vi "Delete old files.vi"(6 "Delete File Action":T1, 8 "error in (no error)":errorcluster, 9 "Entire hierachy (F)":bool, 10 "Retention":i32, 11 "Directory":string[](array[string])) -> (0 "error out":errorcluster)   [LabVIEW 2017, in "File.lvlib"]
uses:
  File.lvlib
  Control/Delete File Action.ctl
  Control/Parent path.ctl
  Error Handler/Error.lvlib
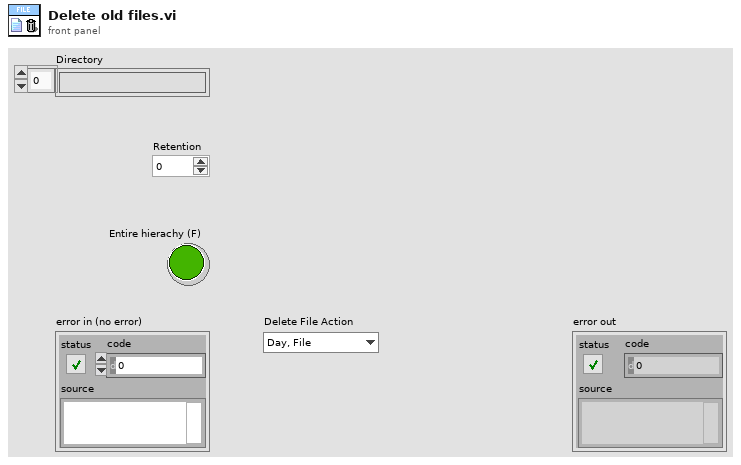
[diagram p1: front panel]
types:
  T1 = typedef "File.lvlib/Delete File Action.ctl" = enum16{"Day, File", "Day, Folder", "Month, File", "Month, Folder"}
  T2 = cluster{"Retention":i32, "Directory":string[], "Entire hierachy (F)":bool, "current time":timestamp}
  T3 = typedef "File.lvlib/Parent path.ctl" = enum16{"Project", "Setting", "Log"}
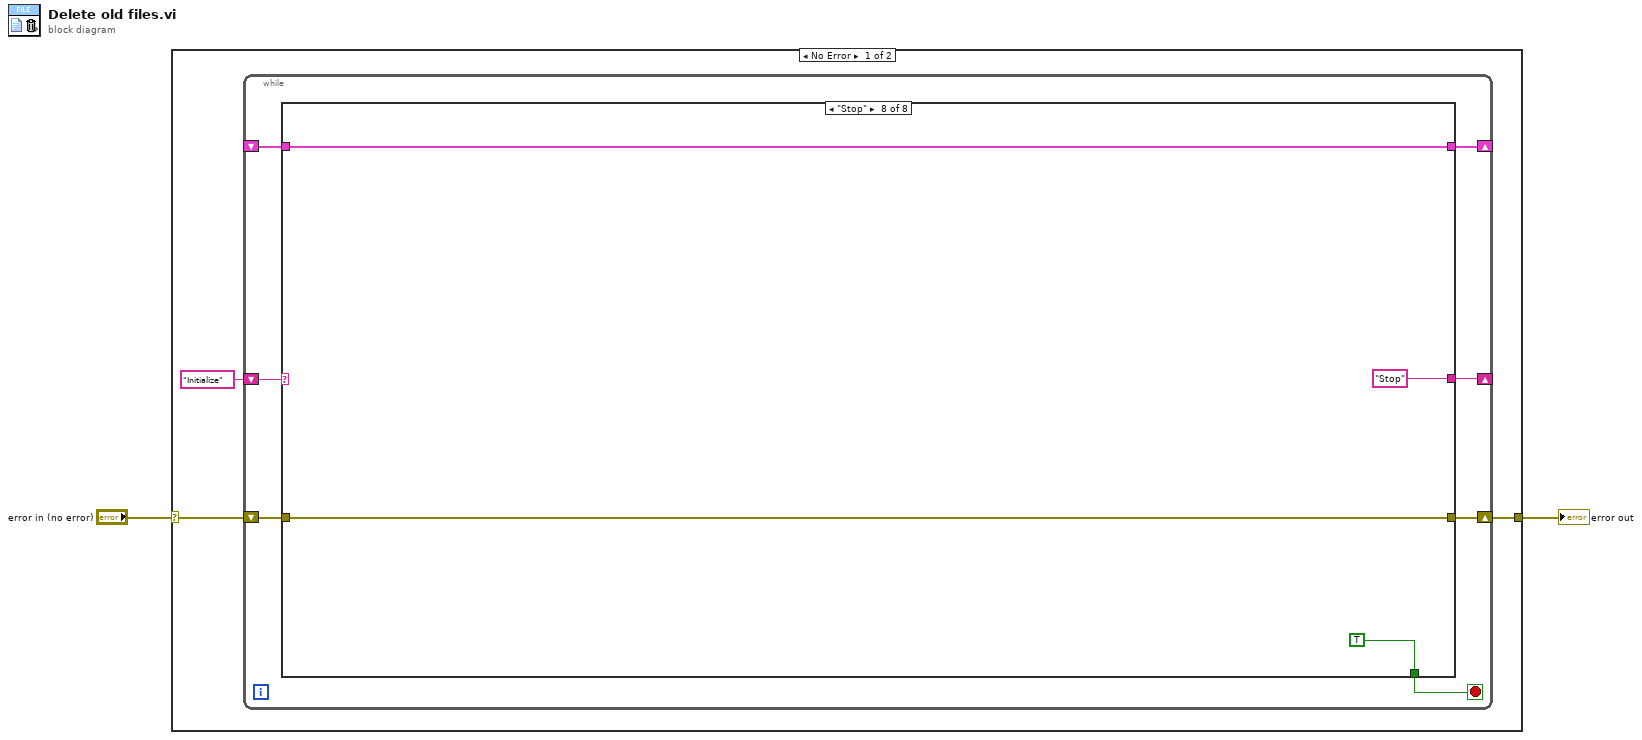
[diagram p0: block diagram]
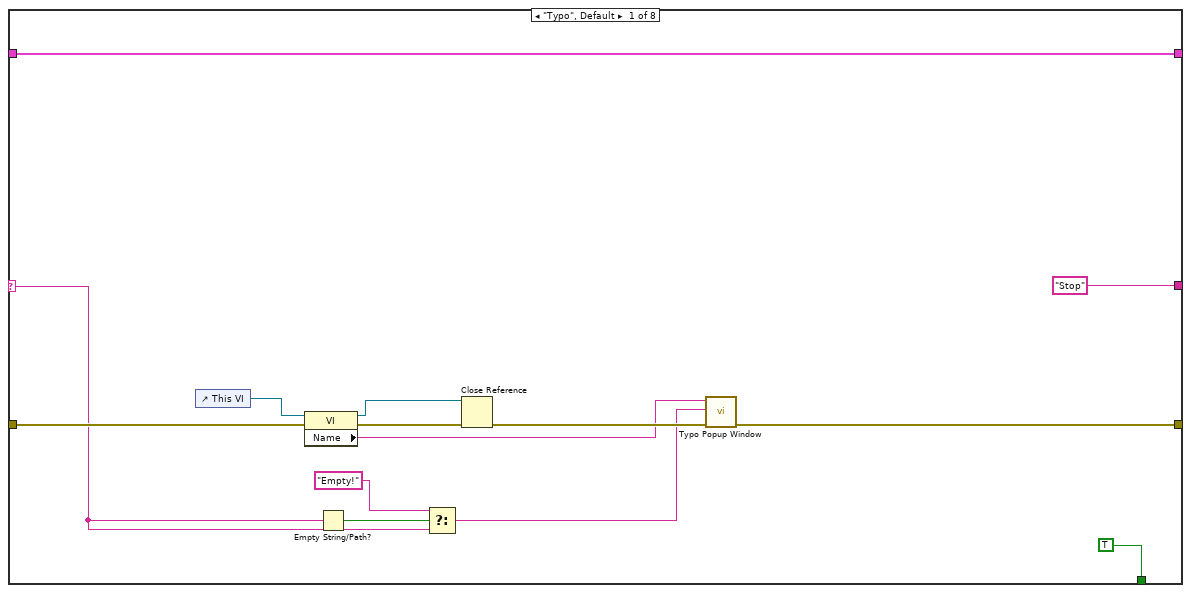
[diagram p2: hidden frame]
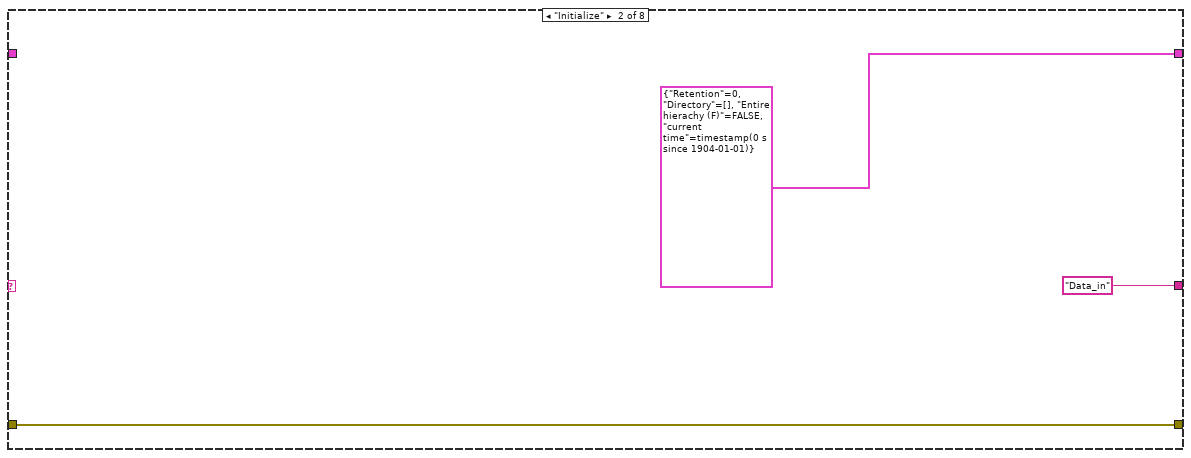
[diagram p3: hidden frame]
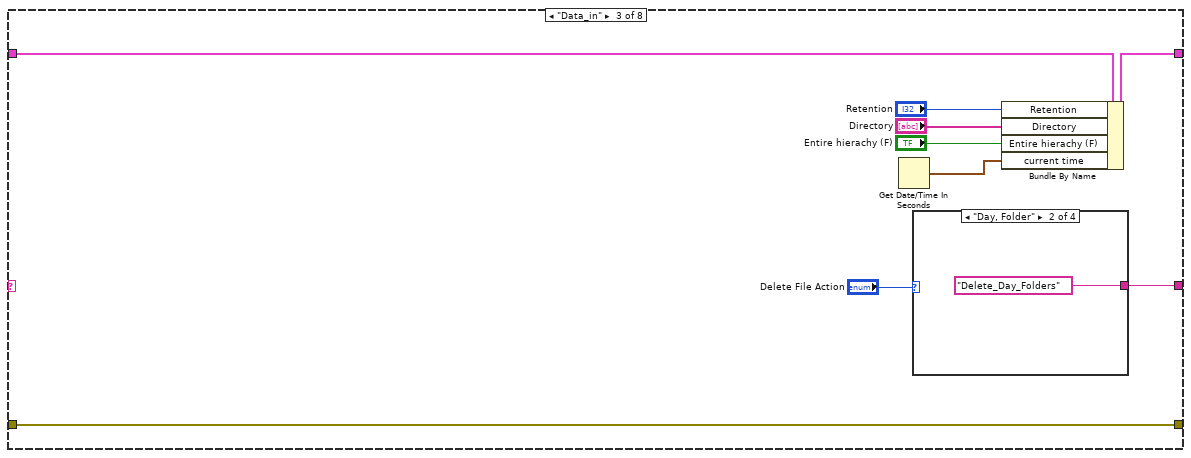
[diagram p4: hidden frame]
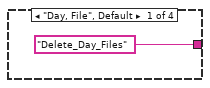
[diagram p5: hidden frame]
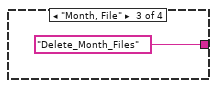
[diagram p6: hidden frame]
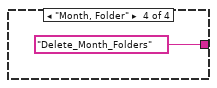
[diagram p7: hidden frame]
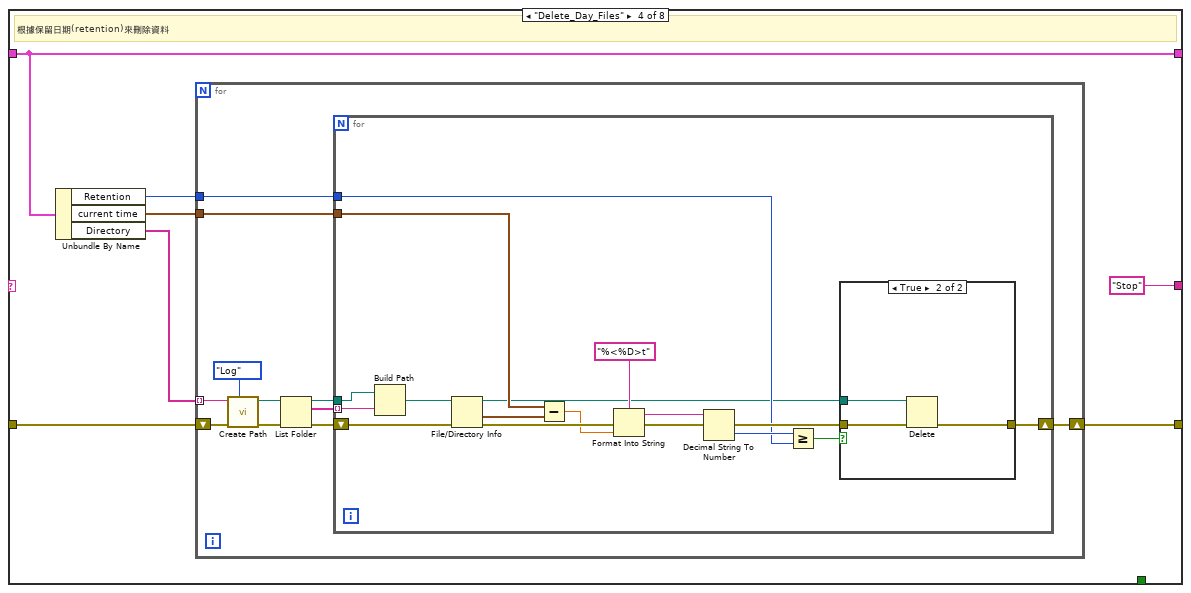
[diagram p8: hidden frame]
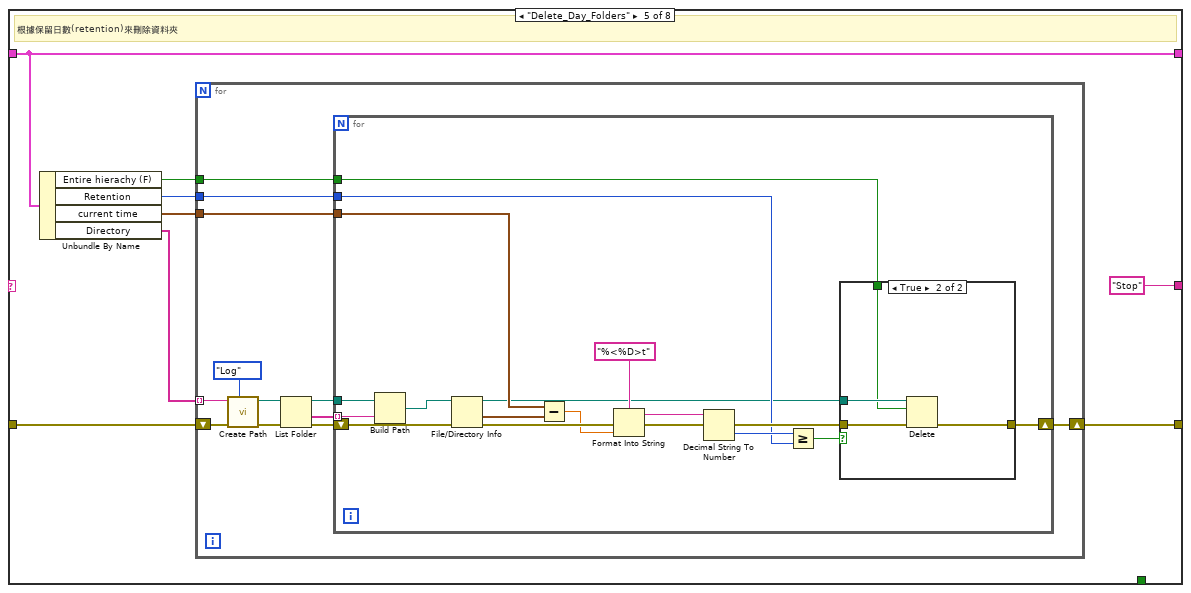
[diagram p10: hidden frame]
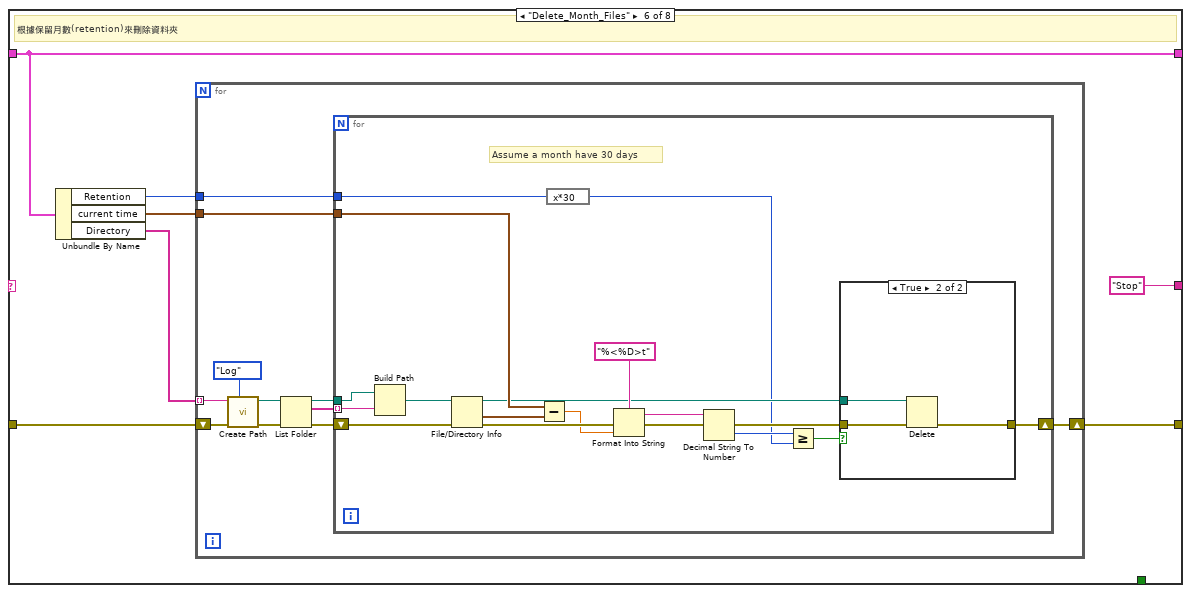
[diagram p12: hidden frame]
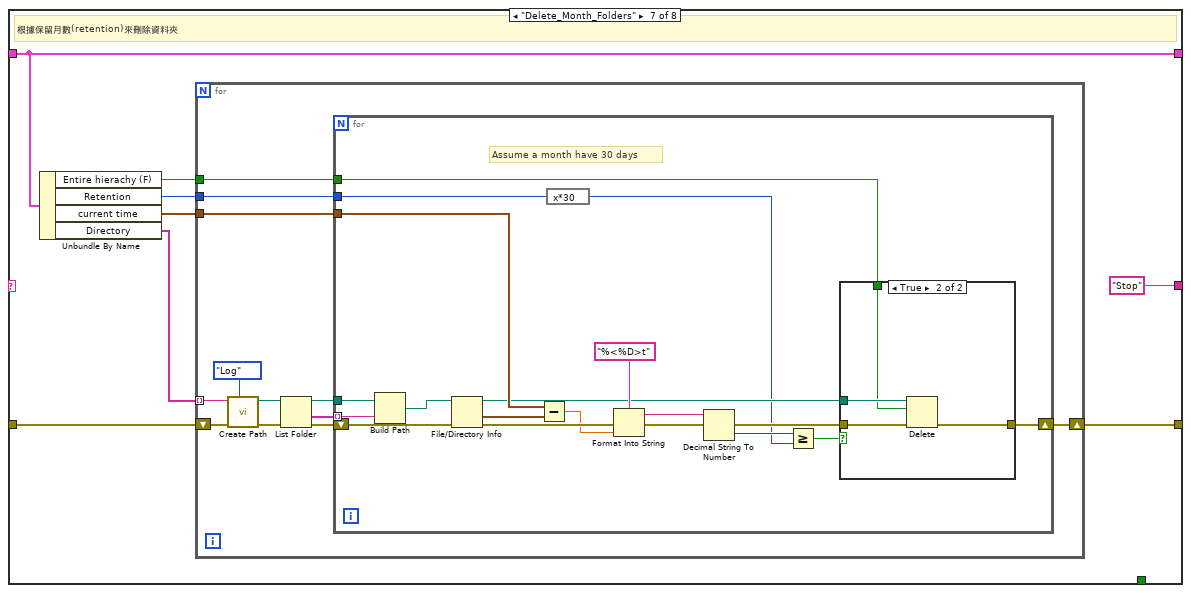
[diagram p14: hidden frame]
diagram:
  n1 = case shown="No Error" "error in (no error)" {
    selector: "error in (no error)" -> [w4 w209]
    tunnel: [w3 w209] -> w1
    frame No Error {
      n2 = while {
        shift-right: [w9] -> _
        shift-left: "Initialize" -> [w12]
        shift-right: [w10] -> w3
        shift-left: w4 -> [w11]
        shift-right: [w7] -> _
        shift-left: _ -> [w6]
        stop <- w8 stop-if-true
        n3 = case shown="\"Stop\"" w12 {
          selector: w12 -> [w20 _ _ _ _ _ _ _]
          tunnel: w11 -> [w26 w29 w38 w49 w88 w129 w169 w208]
          tunnel: [w15 w29 w38 w48 w87 w128 w168 w208] -> w10
          tunnel: ["Stop" "Data_in" w30 "Stop" "Stop" "Stop" "Stop" "Stop"] -> w9
          tunnel: [TRUE _ _ _ _ _ _ TRUE] -> w8
          tunnel: [w16 T2 {"Retention"=0, "Directory"=[], "Entire hierachy (F)"=FALSE, "current time"=timestamp(0 s since 1904-01-01)} w36 w47 w86 w127 w167 w207] -> w7
          tunnel: w6 -> [w16 _ w37 w47 w86 w127 w167 w207]
          frame "Typo", Default {
            n4 = control-ref of="This VI"() -> (w24:refnum<vi>)
            n5 = property class="VI"(reference=w24, error in=w26) -> (reference out=w22:refnum<vi>, error out=w25:errorcluster, "Name"=w14:string)
            n6 = Empty String/Path?(string/path=w20) -> (empty?=w21:bool)
            n7 = Select(t="Empty!", s=w21, f=w20) -> (s? t:f=w13:string)
            n8 = Close Reference(reference=w22, error in (no error)=w25) -> (error out=w23:errorcluster)
            n9 = call "Typo Popup Window.vi"("error in (no error)"=w23, "Typo in"=w13, "VI/Loop name"=w14) -> ("error out"=w15:errorcluster)  [unwired: 8 in]
          }
          frame "Initialize" {
          }
          frame "Data_in" {
            n10 = Get Date/Time In Seconds() -> (seconds since 1Jan1904=w32:timestamp)
            n11 = case shown="\"Day, Folder\"" "Delete File Action" {
              tunnel: ["Delete_Day_Files" "Delete_Day_Folders" "Delete_Month_Files" "Delete_Month_Folders"] -> w30
              frame "Day, File", Default {
              }
              frame "Day, Folder" {
              }
              frame "Month, File" {
              }
              frame "Month, Folder" {
              }
            }
            n12 = Bundle By Name(cluster=w37, "Retention"="Retention", "Directory"="Directory", "Entire hierachy (F)"="Entire hierachy (F)", "current time"=w32) -> (w36:T2)
          }
          frame "Delete_Day_Files" {
            # "根據保留日期(retention)來刪除資料"
            n13 = Unbundle By Name(w47) -> ("Retention"=w44:i32, "current time"=w45:timestamp, "Directory"=w46:string[])
            n14 = for {
              shift-right: [w55] -> w48
              shift-left: w49 -> [w60]
              tunnel: w46 -> [w56] mode=indexing
              tunnel: w45 -> [w52]
              tunnel: w44 -> [w51]
              n15 = call "Create Path.vi"("Parent path"=Parent_path."Log", "error in (no error)"=w60, "Directory"=w56) -> ("error out"=w59:errorcluster, "Path"=w57:path)  [unwired: 7 in]
              n16 = List Folder(path=w57, error in=w59) -> (path out=w54:path, filenames=w53:string[], error out=w58:errorcluster)  [unwired: 2 in, 1 out]
              n17 = for {
                shift-right: [w75] -> w55
                shift-left: w58 -> [w76]
                tunnel: w54 -> [w74]
                tunnel: w53 -> [w73] mode=indexing
                tunnel: w52 -> [w70]
                tunnel: w51 -> [w63]
                n18 = Build Path(base path=w74, name or relative path=w73) -> (appended path=w71:path)
                n19 = File/Directory Info(path=w71, error in=w76) -> (path out=w61:path, last mod=w69:timestamp, error out=w72:errorcluster)  [unwired: 4 out]
                n20 = Subtract(x=w70, y=w69) -> (x-y=w67:dbl)
                n21 = Format Into String(format string="%<%D>t", error in=w72, w67) -> (resulting string=w65:string, error out=w68:errorcluster)  [unwired: 1 in]
                n22 = Decimal String To Number(string=w65) -> (number=w64:i32)  [unwired: 2 in, 1 out]
                n23 = Greater Or Equal?(x=w64, y=w63) -> (x >= y?=w62:bool)
                n24 = case shown="True" w62 {
                  tunnel: w68 -> [w77 w80]
                  tunnel: [w77 w79] -> w75
                  tunnel: w61 -> [_ w78]
                  frame False {
                  }
                  frame True {
                    n25 = Delete(path (use dialog)=w78, error in=w80) -> (error out=w79:errorcluster)  [unwired: 3 in, 2 out]
                  }
                }
              }
            }
          }
          frame "Delete_Day_Folders" {
            # "根據保留日數(retention)來刪除資料夾"
            n26 = Unbundle By Name(w86) -> ("Entire hierachy (F)"=w81:bool, "Retention"=w83:i32, "current time"=w84:timestamp, "Directory"=w85:string[])
            n27 = for {
              shift-right: [w95] -> w87
              shift-left: w88 -> [w100]
              tunnel: w85 -> [w96] mode=indexing
              tunnel: w84 -> [w93]
              tunnel: w83 -> [w92]
              tunnel: w81 -> [w91]
              n28 = call "Create Path.vi"("Parent path"=Parent_path."Log", "error in (no error)"=w100, "Directory"=w96) -> ("error out"=w99:errorcluster, "Path"=w97:path)  [unwired: 7 in]
              n29 = List Folder(path=w97, error in=w99) -> (path out=w94:path, folder names=w90:string[], error out=w98:errorcluster)  [unwired: 2 in, 1 out]
              n30 = for {
                shift-right: [w116] -> w95
                shift-left: w98 -> [w117]
                tunnel: w94 -> [w115]
                tunnel: w93 -> [w112]
                tunnel: w92 -> [w105]
                tunnel: w91 -> [w102]
                tunnel: w90 -> [w101] mode=indexing
                n31 = Build Path(base path=w115, name or relative path=w101) -> (appended path=w113:path)
                n32 = File/Directory Info(path=w113, error in=w117) -> (path out=w103:path, last mod=w111:timestamp, error out=w114:errorcluster)  [unwired: 4 out]
                n33 = Subtract(x=w112, y=w111) -> (x-y=w109:dbl)
                n34 = Format Into String(format string="%<%D>t", error in=w114, w109) -> (resulting string=w107:string, error out=w110:errorcluster)  [unwired: 1 in]
                n35 = Decimal String To Number(string=w107) -> (number=w106:i32)  [unwired: 2 in, 1 out]
                n36 = Greater Or Equal?(x=w106, y=w105) -> (x >= y?=w104:bool)
                n37 = case shown="True" w104 {
                  tunnel: w110 -> [w118 w122]
                  tunnel: [w118 w121] -> w116
                  tunnel: w103 -> [_ w120]
                  tunnel: w102 -> [_ w119]
                  frame False {
                  }
                  frame True {
                    n38 = Delete(path (use dialog)=w120, entire hierarchy (F)=w119, error in=w122) -> (error out=w121:errorcluster)  [unwired: 2 in, 2 out]
                  }
                }
              }
            }
          }
          frame "Delete_Month_Files" {
            # "根據保留月數(retention)來刪除資料夾"
            n39 = Unbundle By Name(w127) -> ("Retention"=w124:i32, "current time"=w125:timestamp, "Directory"=w126:string[])
            n40 = for {
              shift-right: [w135] -> w128
              shift-left: w129 -> [w140]
              tunnel: w126 -> [w136] mode=indexing
              tunnel: w125 -> [w132]
              tunnel: w124 -> [w131]
              n41 = call "Create Path.vi"("Parent path"=Parent_path."Log", "error in (no error)"=w140, "Directory"=w136) -> ("error out"=w139:errorcluster, "Path"=w137:path)  [unwired: 7 in]
              n42 = List Folder(path=w137, error in=w139) -> (path out=w134:path, filenames=w133:string[], error out=w138:errorcluster)  [unwired: 2 in, 1 out]
              n43 = for {
                shift-right: [w156] -> w135
                shift-left: w138 -> [w157]
                tunnel: w134 -> [w155]
                tunnel: w133 -> [w154] mode=indexing
                tunnel: w132 -> [w151]
                tunnel: w131 -> [w144]
                # "Assume a month have 30 days"
                n44 = Build Path(base path=w155, name or relative path=w154) -> (appended path=w152:path)
                n45 = File/Directory Info(path=w152, error in=w157) -> (path out=w142:path, last mod=w150:timestamp, error out=w153:errorcluster)  [unwired: 4 out]
                n46 = Subtract(x=w151, y=w150) -> (x-y=w148:dbl)
                n47 = expression code="x*30"(w144) -> (w141:i32)
                n48 = Format Into String(format string="%<%D>t", error in=w153, w148) -> (resulting string=w146:string, error out=w149:errorcluster)  [unwired: 1 in]
                n49 = Decimal String To Number(string=w146) -> (number=w145:i32)  [unwired: 2 in, 1 out]
                n50 = Greater Or Equal?(x=w145, y=w141) -> (x >= y?=w143:bool)
                n51 = case shown="True" w143 {
                  tunnel: w149 -> [w158 w161]
                  tunnel: [w158 w160] -> w156
                  tunnel: w142 -> [_ w159]
                  frame False {
                  }
                  frame True {
                    n52 = Delete(path (use dialog)=w159, error in=w161) -> (error out=w160:errorcluster)  [unwired: 3 in, 2 out]
                  }
                }
              }
            }
          }
          frame "Delete_Month_Folders" {
            # "根據保留月數(retention)來刪除資料夾"
            n53 = Unbundle By Name(w167) -> ("Entire hierachy (F)"=w162:bool, "Retention"=w164:i32, "current time"=w165:timestamp, "Directory"=w166:string[])
            n54 = for {
              shift-right: [w176] -> w168
              shift-left: w169 -> [w181]
              tunnel: w166 -> [w177] mode=indexing
              tunnel: w165 -> [w174]
              tunnel: w164 -> [w173]
              tunnel: w162 -> [w172]
              n55 = call "Create Path.vi"("Parent path"=Parent_path."Log", "error in (no error)"=w181, "Directory"=w177) -> ("error out"=w180:errorcluster, "Path"=w178:path)  [unwired: 7 in]
              n56 = List Folder(path=w178, error in=w180) -> (path out=w175:path, folder names=w171:string[], error out=w179:errorcluster)  [unwired: 2 in, 1 out]
              n57 = for {
                shift-right: [w198] -> w176
                shift-left: w179 -> [w199]
                tunnel: w175 -> [w197]
                tunnel: w174 -> [w194]
                tunnel: w173 -> [w187]
                tunnel: w172 -> [w184]
                tunnel: w171 -> [w182] mode=indexing
                # "Assume a month have 30 days"
                n58 = Build Path(base path=w197, name or relative path=w182) -> (appended path=w195:path)
                n59 = File/Directory Info(path=w195, error in=w199) -> (path out=w185:path, last mod=w193:timestamp, error out=w196:errorcluster)  [unwired: 4 out]
                n60 = Subtract(x=w194, y=w193) -> (x-y=w191:dbl)
                n61 = expression code="x*30"(w187) -> (w183:i32)
                n62 = Format Into String(format string="%<%D>t", error in=w196, w191) -> (resulting string=w189:string, error out=w192:errorcluster)  [unwired: 1 in]
                n63 = Decimal String To Number(string=w189) -> (number=w188:i32)  [unwired: 2 in, 1 out]
                n64 = Greater Or Equal?(x=w188, y=w183) -> (x >= y?=w186:bool)
                n65 = case shown="True" w186 {
                  tunnel: w192 -> [w200 w204]
                  tunnel: [w200 w203] -> w198
                  tunnel: w185 -> [_ w202]
                  tunnel: w184 -> [_ w201]
                  frame False {
                  }
                  frame True {
                    n66 = Delete(path (use dialog)=w202, entire hierarchy (F)=w201, error in=w204) -> (error out=w203:errorcluster)  [unwired: 2 in, 2 out]
                  }
                }
              }
            }
          }
          frame "Stop" {
          }
        }
      }
    }
    frame Error {
    }
  }
  "error out" <- w1
